vi "Create Stream.vi"(8 "error in (no error)":errorcluster, 10 "IP":string="//localhost", 11 "Channel GUI in":refnum<class "Channel GUI.lvclass">) -> (0 "error out":errorcluster, 3 "Channel GUI out":refnum<class "Channel GUI.lvclass">)   [LabVIEW 2018, in "Channel GUI.lvclass"]
uses:
  Channel GUI.lvclass
  Channel GUI.lvclass/Channel GUI.ctl
  Stream/Stream.lvclass
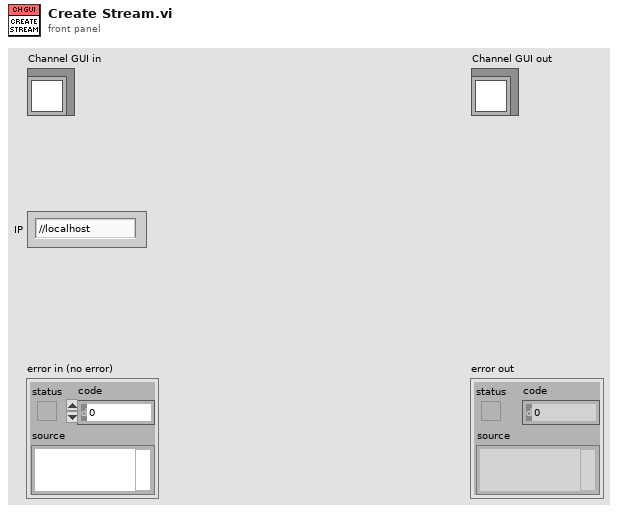
[diagram p1: front panel]
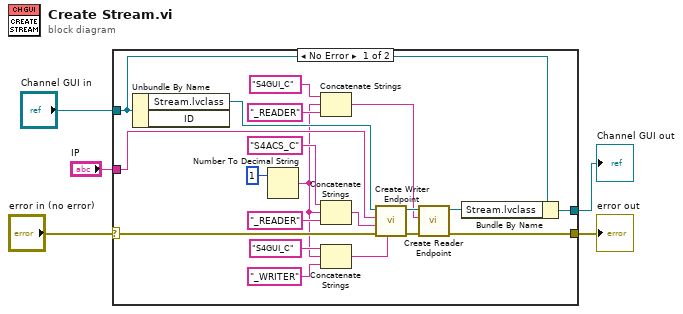
[diagram p0: block diagram]
diagram:
  n1 = case shown="No Error" "error in (no error)" {
    selector: "error in (no error)" -> [w21 w27]
    tunnel: [w22 w27] -> w4
    tunnel: [w19 w26] -> w2
    tunnel: "Channel GUI in" -> [w20 w26]
    tunnel: "IP" -> [w17 _]
    frame No Error {
      n2 = Unbundle By Name(w20) -> ("Stream.lvclass"=w23:refnum<class "Stream.lvclass">)  [unwired: 1 out]
      n3 = Number To Decimal String(number=1) -> (decimal integer string=w9:string)  [unwired: 1 in]
      n4 = Concatenate Strings("S4GUI_C" ("reader name"), w9, "_READER" ("reader name")) -> (w7:string)
      n5 = Concatenate Strings("S4ACS_C" ("reader name"), w9, "_READER" ("reader name")) -> (w12:string)
      n6 = Concatenate Strings("S4GUI_C", w9, "_WRITER") -> (w8:string)
      n7 = call "Create Writer Endpoint.vi"("writer name"=w8, "error in (no error)"=w21, "reader name"=w12, "IP"=w17, "Stream in"=w23) -> ("error out"=w25:errorcluster, "Stream out"=w24:refnum<class "Stream.lvclass">)  [unwired: 5 in]
      n8 = call "Create Reader Endpoint.vi"("error in (no error)"=w25, "reader name"=w7, "Stream in"=w24) -> ("error out"=w22:errorcluster, "Stream out"=w18:refnum<class "Stream.lvclass">)  [unwired: 7 in]
      n9 = Bundle By Name(cluster=w20, "Stream.lvclass"=w18) -> (w19:refnum<class "Channel GUI.lvclass">)
    }
    frame Error {
    }
  }
  "error out" <- w4
  "Channel GUI out" <- w2
